vi "I2C SDA Out(David Documentation).vi"(4 "Clear?":bool, 5 "Address In":u8, 6 "Set?":bool, 7 "Data In":u8, 9 "Setup?":bool, 10 "Load?":bool, 11 "Address?":bool) -> (3 "SDA_OUT":bool)   [LabVIEW 2015]
doc: "This VI configures the SDA Out. See the table in the Block Diagram.\n\nAlso, it holds for 2 clock cycles = 50 ns."
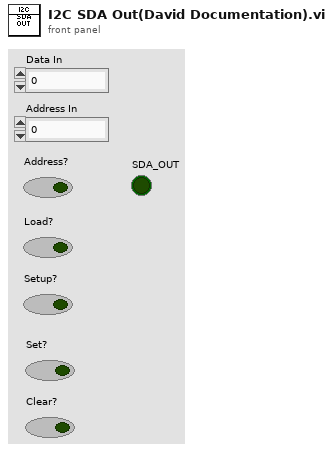
[diagram p1: front panel]
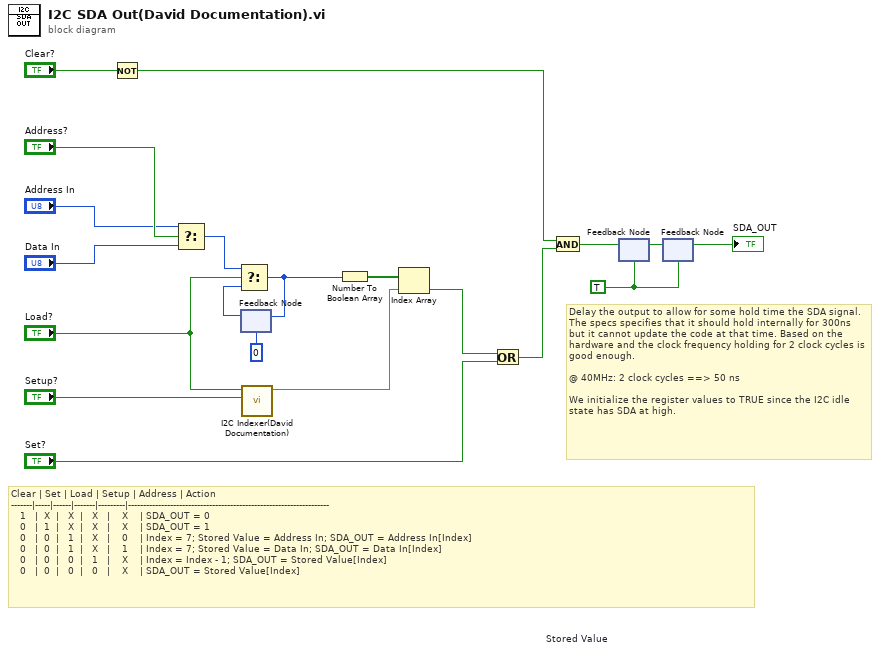
[diagram p0: block diagram]
diagram:
  w1 = TRUE
  # "Delay the output to allow for some hold time the SDA signal. The specs specifies that it should hold internally for 300ns but it cannot update the code at that time. Based on the hardware and the clock frequency holding for 2 clock cycles is good enough. \n\n@ 40MHz: 2 clock cycles ==> 50 ns\n\nWe initialize the register values to TRUE since the I2C idle state has SDA at high."
  # "Clear | Set | Load | Setup | Address | Action\n-------|-----|------|-------|---------|-------------------------------------------------------------------\n   1   |  X  |   X  |   X   |    X    | SDA_OUT = 0\n   0   |  1  |   X  |   X   |    X    | SDA_OUT = 1\n   0   |  0  |   1  |   X   |    0    | Index = 7; Stored Value = Address In; SDA_OUT = Address In[Index]\n   0   |  0  |   1  |   X   |    1    | Index = 7; Stored Value = Data In; SDA_OUT = Data In[Index]\n   0   |  0  |   0  |   1   |    X    | Index = Index - 1; SDA_OUT = Stored Value[Index]\n   0   |  0  |   0  |   0   |    X    | SDA_OUT = Stored Value[Index]"
  n1 = Not(x="Clear?") -> (.not. x?=w12:bool)
  n2 = Select(t="Address In", s="Address?", f="Data In") -> (s? t:f=w19:u8)
  n3 = feedback #1 "Stored Value"(u8 0 ("Address In")) -> (w18:u8)
  n4 = Select(t=w19, s="Load?", f=w18) -> (s? t:f=w17:u8)
  n5 = feedback-in #1(w17) -> ()
  n6 = call "I2C Indexer(David Documentation).vi"("Decrement?"="Setup?", "Load?"="Load?") -> ("Numeric"=w6:fxp<+,3,3>)  [unwired: 9 in]
  n7 = Number To Boolean Array(number=w17) -> (Boolean array=w16:bool[])
  n8 = Index Array(array=w16, index=w6) -> (element=w10:bool)
  n9 = Or(x=w10, y="Set?") -> (x .or. y?=w9:bool)
  n10 = And(x=w12, y=w9) -> (x .and. y?=w11:bool)
  n11 = feedback-in #2(w11) -> ()
  n12 = feedback #2(w1) -> (w3:bool)
  n13 = feedback-in #3(w3) -> ()
  n14 = feedback #3(w1) -> (→"SDA_OUT":bool)
